vi "CCD Configuration.vi"(8 "error in (no error)":errorcluster caption="错误输入（无错误）") -> (0 "error out":errorcluster caption="错误输出", 3 "CCD Configuration":T1)   [LabVIEW 2015, in "CCD.lvlib"]
doc: "该模板用于创建子VI。"
uses:
  CCD.lvlib
  Support/CCD Configuration.ctl
  <vilib>/userdefined/High Color/IMAQdx.ctl
  <vilib>/vision/Image Controls.llb/IMAQ Image.ctl
  Utility VIs/Utility VIs.lvlib
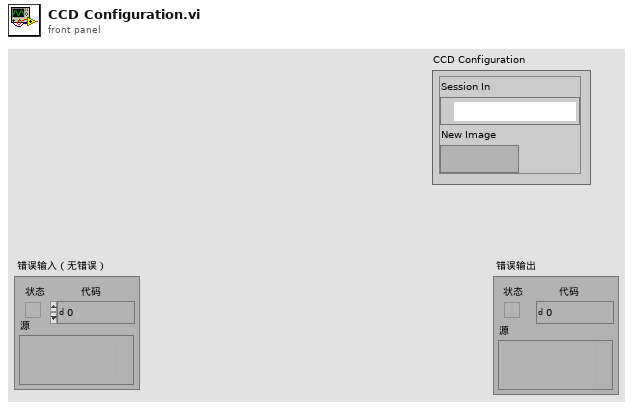
[diagram p1: front panel]
types:
  T1 = typedef "CCD.lvlib/CCD Configuration.ctl" = cluster{"Session In":T2, "New Image":T3}
  T2 = typedef "IMAQdx.ctl" = refnum<k21>
  T3 = typedef "IMAQ Image.ctl" = refnum<image>
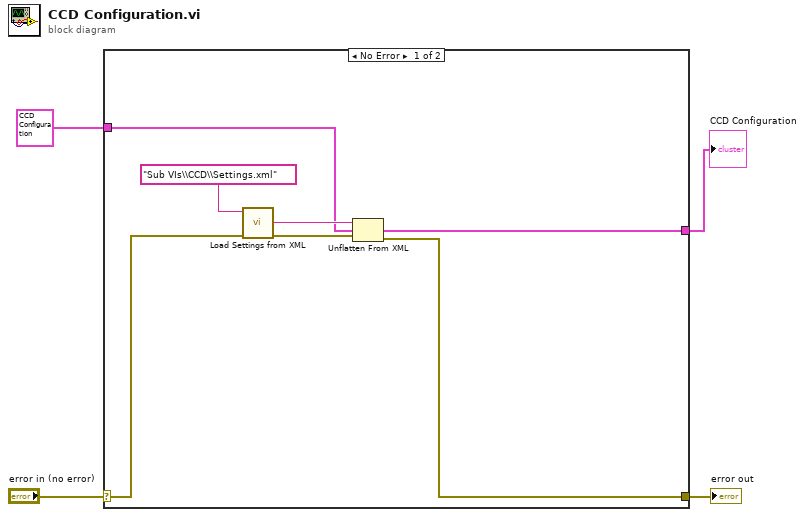
[diagram p0: block diagram]
diagram:
  n1 = case shown="No Error" "error in (no error)" {
    selector: "error in (no error)" -> [w7 w12]
    tunnel: [w6 w12] -> w3
    tunnel: T1 {"Session In"="", "New Image"=refnum} ("CCD Configuration") -> [w9 _]
    tunnel: [w5 _] -> w2
    frame No Error {
      n2 = call "Load Settings from XML.vi"("error in (no error)"=w7, "名称或相对路径"="Sub VIs\\CCD\\Settings.xml") -> ("error out"=w8:errorcluster, "XML Elements"=w10:string)  [unwired: 8 in]
      n3 = Unflatten From XML(xml string=w10, type=w9, error in (no error)=w8) -> (value=w5:T1, error out=w6:errorcluster)
    }
    frame Error {
    }
  }
  "error out" <- w3
  "CCD Configuration" <- w2
